vi "Robot Global Data.vi"() -> ()   [LabVIEW 2017]
doc: "This global VI can contain as many global variables as you need. Place a control on the panel, give it a good name. To read or write to it from a VI, drag the icon to the diagram of that VI. You can also drag from the project. Click on the node to change which global you access. You shouldn't have multiple locations writing to a global or it will cause a race-condition."
uses:
  <vilib>/Rock Robotics/WPI/Camera/WPI_CameraImageSize.ctl
  LabVIEW_is_Under_Control.lib/Util/Unpack Gamepad/Axes Cluster.ctl
  LabVIEW_is_Under_Control.lib/Util/Unpack Gamepad/Button Cluster.ctl
  <vilib>/Rock Robotics/WPI/DriverStation/WPI_DriverStationRobotMode2.ctl
  LabVIEW_is_Under_Control.lib/Util/Unpack Gamepad/D-Pad.ctl
panel:
  out "Scale_side":string
  out "Switch_side":string
  in  "Starting Conf. Override":bool
  in  "2Cube Auto":bool
  in  "4bar Override":bool
  in  "Speed Override":bool
  in  "Gear Override":bool
  in  "Elevator_Override":bool
  in  "Exchange_Height":dbl
  in  "Kf":dbl=1.0
  in  "Reset Yaw + Encoders":bool
  out "D-Pad":T1
  in  "Elevador_Setpoint":dbl
  in  "Elevador_Height":dbl
  in  "Reset_Elevador":bool
  in  "AutoForward":bool
  in  "Right Tração Value":dbl
  in  "Left Tração Value":dbl
  in  "Yaw":dbl
  in  "EncoderTraçaoEsq":dbl
  in  "EncoderTraçaoDir":dbl
  in  "Throttle  auto":dbl
  in  "Wheel auto":dbl
  in  "Gear Value":bool
  in  "4Bar Value":bool
  in  "Intake IR Value":bool
  in  "Intake Motor Value":dbl
  in  "Robot Mode":T2
  in  "Xbox2 Axes":T3
  out "Xbox2 Buttons":T4
  out "Xbox Buttons":T4
  in  "Xbox Axes":T3
  in  "image size":T5=enum."320x240"
  in  "Enable Vision":bool
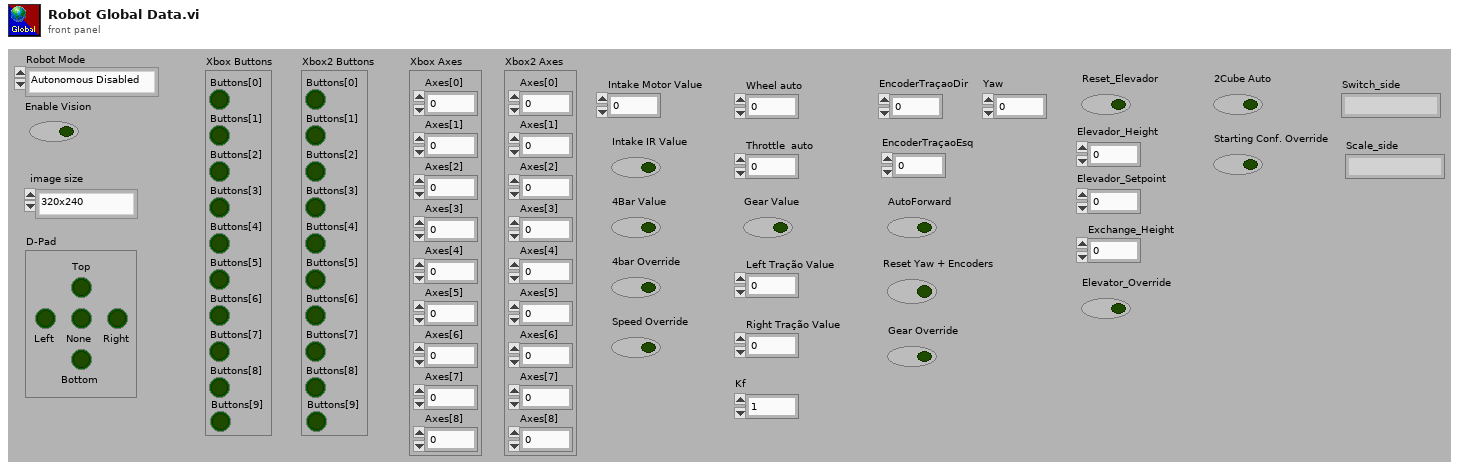
[diagram p1: front panel]
types:
  T1 = typedef "D-Pad.ctl" = cluster{"Top":bool, "Bottom":bool, "None":bool, "Right":bool, "Left":bool}
  T2 = typedef "WPI_DriverStationRobotMode2.ctl" = enum16{"Autonomous Disabled", "Autonomous Enabled", "Teleop Disabled", "Teleop Enabled", "Disconnected", "Finish", "Test Disabled", "Test Enabled", "Emergency Stopped"}
  T3 = typedef "Axes Cluster.ctl" = cluster{"Axes[0]":dbl, "Axes[1]":dbl, "Axes[2]":dbl, "Axes[3]":dbl, "Axes[4]":dbl, "Axes[5]":dbl, "Axes[6]":dbl, "Axes[7]":dbl, "Axes[8]":dbl}
  T4 = typedef "Button Cluster.ctl" = cluster{"Buttons[0]":bool, "Buttons[1]":bool, "Buttons[2]":bool, "Buttons[3]":bool, "Buttons[4]":bool, "Buttons[5]":bool, "Buttons[6]":bool, "Buttons[7]":bool, "Buttons[8]":bool, "Buttons[9]":bool}
  T5 = typedef "WPI_CameraImageSize.ctl" = enum16{"640x480", "320x240", "160x120", "Custom"}
diagram:
